vi "Max Bandwidth.vi"(1 "resources":i32[](array[numeric])) -> (0 "disabled ranges":i32[](array[numeric]))   [LabVIEW 2022 SP3, in "EClib functions.lvlib"]
doc: "Builds an arrays of indices of the unavailable bandwidth values."
uses:
  EClib functions.lvlib
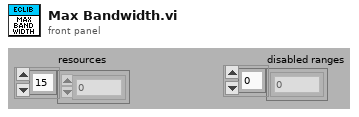
[diagram p1: front panel]
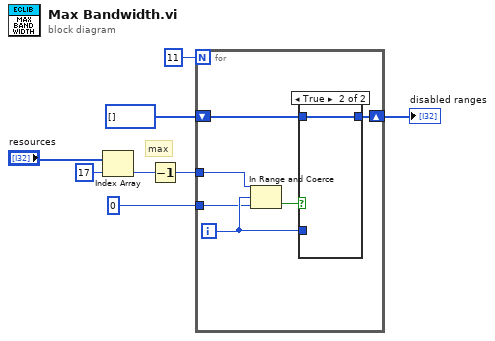
[diagram p0: block diagram]
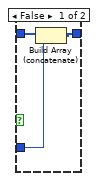
[diagram p2: hidden frame]
diagram:
  # "max"
  n1 = Index Array(array="resources", index=17) -> (element=w2:i32)
  n2 = Decrement(x=w2) -> (x-1=w1:i32)
  n3 = for {
    N: 11 -> [_]
    tunnel: w1 -> [w14]
    shift-right: [w12] -> w4
    shift-left: i32[] [] -> [w11]
    tunnel: 0 ("limite basse") -> [w9]
    i -> [w10]
    n4 = In Range and Coerce(upper limit=w14, x=w10, lower limit=w9) -> (In Range?=w13:bool)  [unwired: 1 out]
    n5 = case shown="True" w13 {
      tunnel: w10 -> [w17 _]
      tunnel: [w16 w18] -> w12
      tunnel: w11 -> [w15 w18]
      frame False {
        n6 = Build Array (concatenate)(w15, w17) -> (w16:i32[])
      }
      frame True {
      }
    }
  }
  "disabled ranges" <- w4
